vi "SEND CAN data FD.vi"() -> ()   [LabVIEW 2016]
doc: "This is a practical example of CAN_WRITE_FD.\nFirst of all the selected channel will be initiatlized.\nOnce the initialisation is OK a timed while loop will be executed until CAN_WRITE_FD will signal an error.\nSince CAN_WRITE_FD isn't limited to eight bytes this example transmitts 9 Bytes.\nYou'll see that the CAN_READ_FD example will show you 12 received byted according to the CAN_FD specification."
uses:
  CAN Communication.llb/TPCANParameter.ctl
  CAN Communication.llb/TPCANHandle.ctl
  CAN Communication.llb/CAN MSG Cluster.ctl
  <vilib>/Platform/TimedLoop/XDataNode/XDataNode.xnode
  <vilib>/Platform/TimedLoop/XDataNode/timing_clust.ctl
  <vilib>/Platform/TimedLoop/XDataNode/XDNodeRunTimeDep.lvlib
  <vilib>/Platform/TimedLoop/XDataNode/wakeup.ctl
  <vilib>/Platform/TimedLoop/XDataNode/nitl_modes.ctl
  CAN Communication.llb/PCAN Get CHANNEL CONDITION.vi
  CAN Communication.llb/PCAN Get CHANNEL IDENTIFYING.vi
  CAN Communication.llb/PCAN Bus Off Auto Reset.ctl
panel:
  out "IDENTIFYING PARAM":T1
  out "error out":errorcluster
  out "input cluster":T2 {"MSG type" format="%x"; "ID" format="%.0x"}
  in  "Release all channels first":bool
  in  "TPCANHandle":T3=enum."PCAN_USBBUS2  0x52"
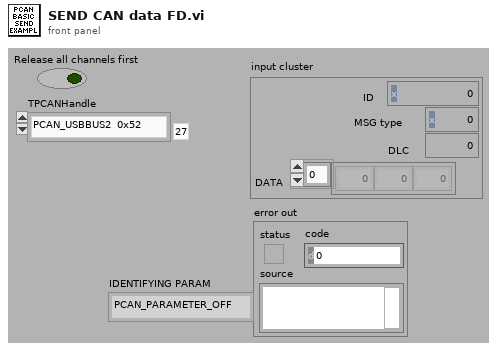
[diagram p1: front panel]
types:
  T1 = typedef "PCAN Bus Off Auto Reset.ctl" = enum32{"PCAN_PARAMETER_OFF", "PCAN_PARAMETER_ON"}
  T2 = typedef "CAN MSG Cluster.ctl" = cluster{"ID":u32, "MSG type":u8, "DLC":u8, "DATA":u8[]}
  T3 = typedef "TPCANHandle.ctl" = enum16{"PCAN_NONEBUS  0x000", "PCAN_ISABUS1  0x21", "PCAN_ISABUS2  0x22", "PCAN_ISABUS3  0x23", "PCAN_ISABUS4  0x24", "PCAN_ISABUS5  0x25", "PCAN_ISABUS6  0x26", "PCAN_ISABUS7  0x27", "PCAN_ISABUS8  0x28", "PCAN_DNGBUS1  0x31", "PCAN_PCIBUS1  0x41", "PCAN_PCIBUS1  0x42", "PCAN_PCIBUS1  0x43", "PCAN_PCIBUS1  0x44", "PCAN_PCIBUS1  0x45", "PCAN_PCIBUS1  0x46", "PCAN_PCIBUS1  0x47", "PCAN_PCIBUS1  0x48", "PCAN_PCIBUS1  0x409", "PCAN_PCIBUS1  0x40A", "PCAN_PCIBUS1  0x40B", "PCAN_PCIBUS1  0x40C", "PCAN_PCIBUS1  0x40D", "PCAN_PCIBUS1  0x40E", "PCAN_PCIBUS1  0x40F", "PCAN_PCIBUS1  0x410", "PCAN_USBBUS1  0x51", "PCAN_USBBUS2  0x52", "PCAN_USBBUS3  0x53", "PCAN_USBBUS4  0x54", "PCAN_USBBUS5  0x55", "PCAN_USBBUS6  0x56", "PCAN_USBBUS7  0x57", "PCAN_USBBUS8  0x58", "PCAN_USBBUS9  0x509", "PCAN_USBBUS10  0x50A", "PCAN_USBBUS11  0x50B", "PCAN_USBBUS12  0x50C", "PCAN_USBBUS13  0x50D", "PCAN_USBBUS14  0x50E", "PCAN_USBBUS15  0x50F", "PCAN_USBBUS16  0x510", "PCAN_PCCBUS1  0x61", "PCAN_PCCBUS2  0x62", "PCAN_LANBUS1  0x801", "PCAN_LANBUS2  0x802", "PCAN_LANBUS3  0x803", "PCAN_LANBUS4  0x804", "PCAN_LANBUS5  0x805", "PCAN_LANBUS6  0x806", "PCAN_LANBUS7  0x807", "PCAN_LANBUS8  0x808", "PCAN_LANBUS9  0x809", "PCAN_LANBUS10  0x80A", "PCAN_LANBUS11  0x80B", "PCAN_LANBUS12  0x80C", "PCAN_LANBUS13  0x80D", "PCAN_LANBUS14  0x80E", "PCAN_LANBUS15  0x80F", "PCAN_LANBUS16  0x810"}
  T4 = typedef "TPCANParameter.ctl" = enum8{"Not Available", "PCAN device number", "PCAN 5-volt power", "PCAN receive event", "PCAN message filter", "PCAN API version", "PCAN channel version", "PCAN busoff autoreset", "PCAN listen-only", "PCAN log location", "PCAN log status", "PCAN log configure", "PCAN log text", "PCAN channel condition", "PCAN hardware name", "PCAN_RECEIVE_STATUS", "PCAN_CONTROLLER_NUMBER", "PCAN_TRACE_LOCATION ", "PCAN_TRACE_STATUS", "PCAN_TRACE_SIZE", "PCAN_TRACE_CONFIGURE", "PCAN_CHANNEL_IDENTIFYING", "PCAN_CHANNEL_FEATURES", "PCAN_SPEED_ADAPTING", "PCAN_BITRATE_INFO", "PCAN_BITRATE_INFO_FD", "PCAN_BUSSPEED_NOMINAL", "PCAN_BUSSPEED_DATA", "PCAN_IP_ADDRESS", "PCAN_LAN_SERVICE_STATUS", "PCAN_ALLOW_STATUS_FRAMES", "PCAN_ALLOW_RTR_FRAMES", "PCAN_ALLOW_ERROR_FRAMES", "PCAN_INTERFRAME_DELAY", "PCAN_ACCEPTANCE_FILTER_11BIT", "PCAN_ACCEPTANCE_FILTER_29BIT", "PCAN_IO_DIGITAL_CONFIGURATION", "PCAN_IO_DIGITAL_VALUE", "PCAN_IO_DIGITAL_SET", "PCAN_IO_DIGITAL_CLEAR", "PCAN_IO_ANALOG_VALUE"}
  T5 = typedef "Channel Availability.ctl" = enum16{"PCAN_CHANNEL_UNAVAILABLE", "PCAN_CHANNEL_AVAILABLE", "PCAN_CHANNEL_OCCUPIED"}
  T6 = typedef "XDNodeRunTimeDep.lvlib/timing_clust.ctl" = cluster{"Expected End [f-1]":u64, "Actual End [f-1]":u64, "Finished Late? [f-1]":bool, "Expected End [i-1]":u64, "Actual End [i-1]":u64, "Finished Late? [i-1]":bool, "Expected Start [i]":u64, "Actual Start [i]":u64, "Expected Start [f]":u64, "Actual Start [f]":u64, "Source Name":string, "Structure Name":string, "Period":i64, "Deadline":i64, "Offset":i64, "Start":i64, "Priority":i32, "Timeout":i32, "Mode":T7, "Wakeup Reason":T8, "Error":errorcluster, "Source Type":string, "Secondary Source Type":string, "Global End Time":u64, "Global Start Time":u64, "Frame Duration":u64, "Iteration Duration":u64, "Assigned CPU":i32, "I/O Scan Engine Mode":u32}
  T7 = typedef "XDNodeRunTimeDep.lvlib/nitl_modes.ctl" = enum32{"No Change", "Process missed periods, maintain original phase", "Discard missed periods, maintain original phase", "Process missed periods, ignore original phase", "Discard missed periods, ignore original phase"}
  T8 = typedef "XDNodeRunTimeDep.lvlib/wakeup.ctl" = enum32{"Normal", "Aborted", "Asynchronous wakeup", "Timing source error", "Timed loop error", "Timeout"}
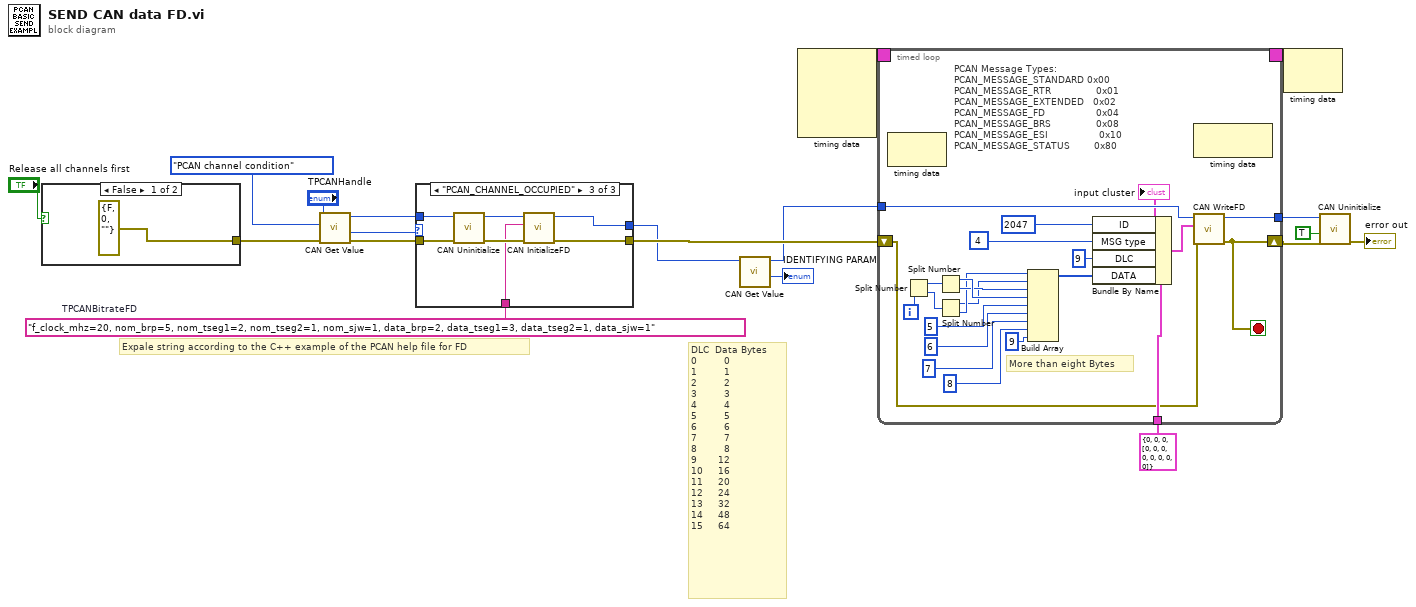
[diagram p0: block diagram]
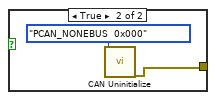
[diagram p2: hidden frame]
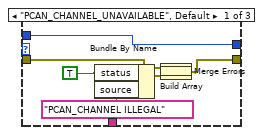
[diagram p3: hidden frame]
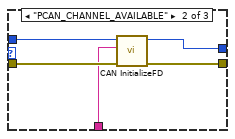
[diagram p4: hidden frame]
diagram:
  w9 = "f_clock_mhz=20, nom_brp=5, nom_tseg1=2, nom_tseg2=1, nom_sjw=1, data_brp=2, data_tseg1=3, data_tseg2=1, data_sjw=1"  # TPCANBitrateFD
  # "DLC  Data Bytes  \n0         0  \n1         1  \n2         2  \n3         3  \n4         4  \n5         5 \n6         6  \n7         7  \n8         8  \n9       12  \n10     16  \n11     20  \n12     24  \n13     32  \n14     48  \n15     64"
  # "Expale string according to the C++ example of the PCAN help file for FD"
  n1 = case shown="False" "Release all channels first" {
    tunnel: [errorcluster {"status"=FALSE, "code"=0, "source"=""} ("error out") w23] -> w15
    frame False {
    }
    frame True {
      n2 = call "CAN Uninitialize.vi"("TPCANHandle"=TPCANHandle."PCAN_NONEBUS  0x000" ("Channel")) -> ("error out"=w23:errorcluster)  [unwired: 8 in, 2 out]
    }
  }
  n3 = call-poly "CAN Get Value.vi"("error in (no error)"=w15, "TPCANParameter"=TPCANParameter."PCAN channel condition" ("Parameter"), "TPCANHandle"="TPCANHandle") -> ("error out"=w17:errorcluster, "Channel condition"=w16:T5, "TPCANHandle out"=w18:T3)  [unwired: 6 in]
  n4 = case shown="\"PCAN_CHANNEL_OCCUPIED\"" w16 {
    tunnel: [w29 w32 w38] -> w11
    tunnel: w18 -> [w30 w34 w41]
    tunnel: w17 -> [w28 w35 w42]
    tunnel: [w30 w33 w39] -> w8
    tunnel: w9 -> [_ w31 w36]
    frame "PCAN_CHANNEL_UNAVAILABLE", Default {
      n5 = Bundle By Name(cluster=w28, "status"=TRUE, "source"="PCAN_CHANNEL ILLEGAL") -> (w25:errorcluster)
      n6 = Build Array(w28, w25) -> (w24:errorcluster[])
      n7 = Merge Errors(w24) -> (w29:errorcluster)
    }
    frame "PCAN_CHANNEL_AVAILABLE" {
      n8 = call "CAN InitializeFD.vi"("error in (no error)"=w35, "TPCANBitrateFD"=w31, "TPCANHandle"=w34) -> ("error out"=w32:errorcluster, "TPCANHandle out"=w33:T3)  [unwired: 5 in, 2 out]
    }
    frame "PCAN_CHANNEL_OCCUPIED" {
      n9 = call "CAN Uninitialize.vi"("error in (no error)"=w42, "TPCANHandle"=w41) -> ("error out"=w37:errorcluster, "TPCANHandle out"=w40:T3)  [unwired: 7 in, 1 out]
      n10 = call "CAN InitializeFD.vi"("error in (no error)"=w37, "TPCANBitrateFD"=w36, "TPCANHandle"=w40) -> ("error out"=w38:errorcluster, "TPCANHandle out"=w39:T3)  [unwired: 5 in, 2 out]
    }
  }
  n11 = call-poly "CAN Get Value.vi"("TPCANHandle"=w8) -> ("error out"=w6:errorcluster, "IDENTIFYING PARAM"=→"IDENTIFYING PARAM":T1, "TPCANHandle out"=w7:T3)  [unwired: 8 in]
  n12 = node-c288() -> (w13:T6)  [unwired: 4 in]
  n13 = timed-loop {
    timing: w13 -> [_]
    timing-out: [_] -> w12
    tunnel: w7 -> [w55]
    tunnel: T2 {"ID"=0, "MSG type"=0, "DLC"=0, "DATA"=[0, 0, 0, 0, 0, 0, 0, 0]} ("CAN_Message") -> [w64]
    shift-right: [w52] -> w3
    shift-left: w11 -> [w53]
    tunnel: [w43] -> w4
    i -> [w62]
    stop <- w52 stop-if-true
    # "PCAN Message Types:\nPCAN_MESSAGE_STANDARD 0x00\nPCAN_MESSAGE_RTR               0x01\nPCAN_MESSAGE_EXTENDED   0x02\nPCAN_MESSAGE_FD                 0x04\nPCAN_MESSAGE_BRS               0x08\nPCAN_MESSAGE_ESI                 0x10\nPCAN_MESSAGE_STATUS        0x80"
    # "More than eight Bytes"
    n14 = node-c288() -> ()  [unwired: 1 in, 1 out]
    n15 = Split Number(x=w62) -> (hi(x)=w60:u16, lo(x)=w61:u16)
    n16 = Split Number(x=w60) -> (hi(x)=w59:u8, lo(x)=w58:u8)
    n17 = Split Number(x=w61) -> (hi(x)=w56:u8, lo(x)=w57:u8)
    n18 = Build Array(w57, w56, w58, w59, u8 5 ("element"), u8 6 ("element"), u8 7 ("element"), u8 8 ("element"), u8 9 ("element")) -> (w51:u8[])
    n19 = Bundle By Name(cluster=w64, "ID"=u32 2047, "MSG type"=u8 4, "DLC"=u8 9, "DATA"=w51) -> (w54:T2)
    "input cluster" <- w54
    n20 = node-c288() -> ()  [unwired: 1 in, 1 out]
    n21 = call "CAN WriteFD.vi"("error in (no error)"=w53, "CAN_Message"=w54, "TPCANHandle"=w55) -> ("error out"=w52:errorcluster, "TPCANHandle out"=w43:T3)  [unwired: 7 in]
  }
  n22 = node-c288(w12) -> ()  [unwired: 1 out]
  n23 = call "CAN Uninitialize.vi"("error in (no error)"=w3, "Ignore input error"=TRUE, "TPCANHandle"=w4) -> ("error out"=→"error out":errorcluster)  [unwired: 6 in, 2 out]
